vi "Resource Monitor.vi"() -> ()   [LabVIEW 2012]
doc: "Shows totals and availability for CPUs, hard drive, and memory resources."
uses:
  <vilib>/Utility/error.llb/DialogType.ctl
  <vilib>/nisyscfg/Close (Hardware).vi
  <vilib>/nisyscfg/Close (System).vi
  <resource>/objmgr/nisysapi.rc
  <vilib>/nisyscfg/nisyscfg.lvlib
panel:
  in  "Polling Interval":u32
  in  "User Name":string
  in  "Password":string
  in  "Target (localhost)":refnum<k21>="localhost"
  in  "stop":bool
  in  "System Properties":enum32{"CPU Usage", "Memory Usage"}(tab)
  out "CPU 0":u32[][](graph)
  out "CPU 2":u32[][](graph)
  out "CPU 3":u32[][](graph)
  out "CPU 1":u32[][](graph)
  out "CPU 4":u32[][](graph)
  out "CPU 5":u32[][](graph)
  out "CPU 6":u32[][](graph)
  out "CPU 7":u32[][](graph)
  out "Number of CPUs":i32
  out "Hard Drive Space Used (%)":dbl(slide) scale=0.0..100.0
  out "Memory":dbl[][](graph)
  out "Primary Hard Drive Available (MB)":dbl
  out "Total Physical Memory (MB)":u32
  out "Total Virtual Memory (MB)":u32
  out "Primary Hard Drive Capacity (MB)":u32
  # "Overview: Shows totals and availability for CPUs, hard drive, and memory resources. \nRequirements: NI System Configuration\nInstructions:\n1. Select your Target. Enter User Name and Password.\n2. Run the VI."
  # "Graphs will automatically populate with the number of cores detected on the computer. For systems with more then eight cores, only the first eight cores will be graphed in this example."
  # "NOTE: If values are 0, then the property is not supported by the specified Target."
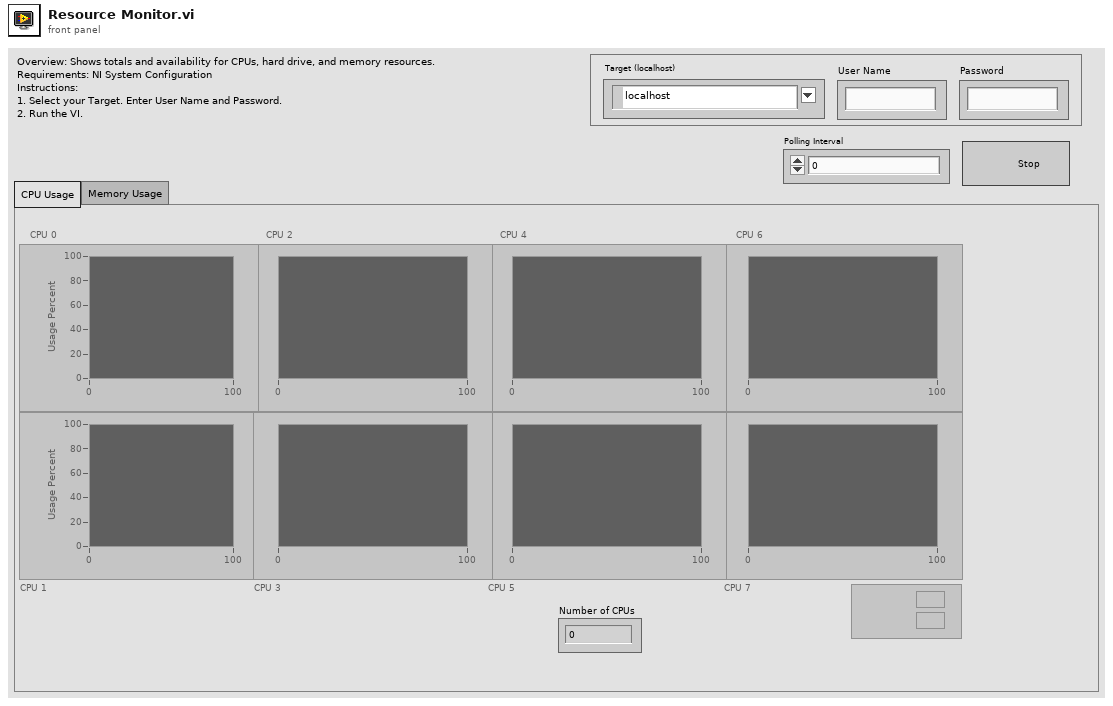
[diagram p1: front panel]
types:
  T1 = typedef "DialogType.ctl" = u16
  T2 = enum8{"Enabled", "Disabled", "Disabled and Grayed Out"}
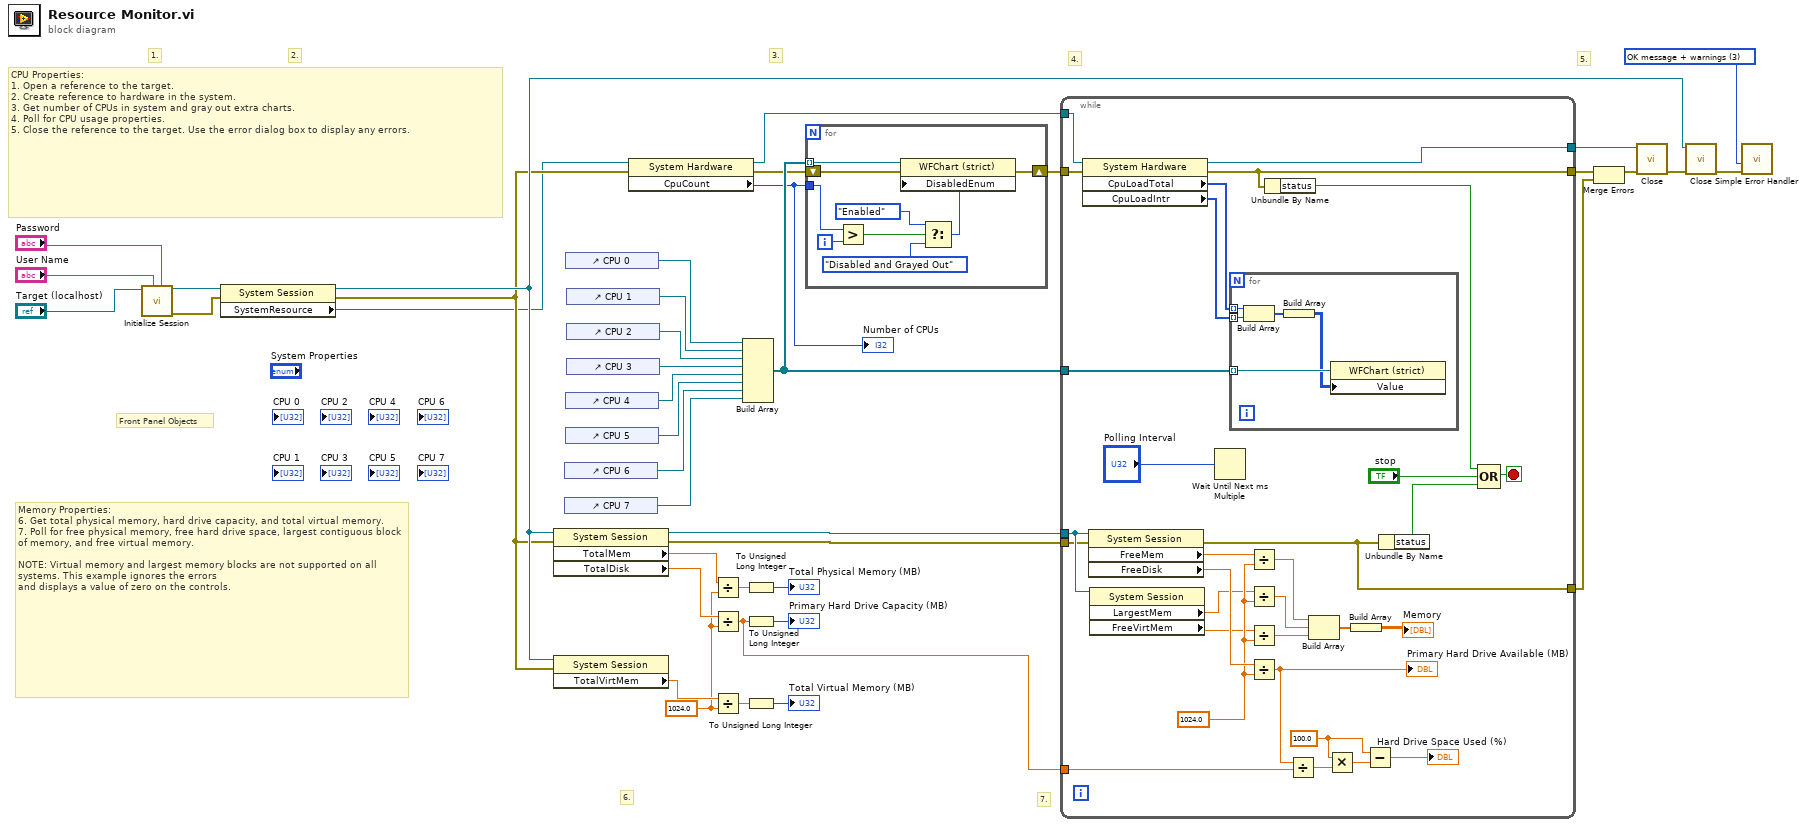
[diagram p0: block diagram]
diagram:
  w15 = T1 3 items=["no dialog", "OK message", "continue or stop message", "OK message + warnings", "continue/stop + warnings"] ("type of dialog (OK msg:1)")
  w23 = 1024.0
  # "2."
  # "Front Panel Objects"
  # "4."
  # "5."
  # "3."
  # "1."
  # "CPU Properties:\n1. Open a reference to the target.\n2. Create reference to hardware in the system.\n3. Get number of CPUs in system and gray out extra charts.\n4. Poll for CPU usage properties.\n5. Close the reference to the target. Use the error dialog box to display any errors."
  # "Memory Properties:\n6. Get total physical memory, hard drive capacity, and total virtual memory.\n7. Poll for free physical memory, free hard drive space, largest contiguous block of memory, and free virtual memory.\n\nNOTE: Virtual memory and largest memory blocks are not supported on all systems. This example ignores the errors\nand displays a value of zero on the controls."
  # "7."
  # "6."
  n1 = call <vilib>:"Initialize Session.vi"("Password"="Password", "User Name"="User Name", "Target (localhost)"="Target (localhost)") -> ("error out"=w8:errorcluster, "Session out"=w9:refnum<k21>)  [unwired: 7 in]
  n2 = property class="System Session"(reference=w9, error in=w8) -> (reference out=w7:refnum<k21>, error out=w6:errorcluster, "SystemResource"=w5:refnum<k20>)
  n3 = property class="System Session"(reference=w7, error in=w6) -> (reference out=w17:refnum<k21>, error out=w13:errorcluster, "TotalMem"=w26:dbl, "TotalDisk"=w25:dbl)
  n4 = property class="System Session"(reference=w7, error in=w6) -> ("TotalVirtMem"=w24:dbl)  [unwired: 2 out]
  n5 = control-ref of="CPU 6"() -> (w34:refnum<vi>)
  n6 = control-ref of="CPU 7"() -> (w27:refnum<vi>)
  n7 = control-ref of="CPU 0"() -> (w4:refnum<vi>)
  n8 = control-ref of="CPU 4"() -> (w36:refnum<vi>)
  n9 = control-ref of="CPU 5"() -> (w35:refnum<vi>)
  n10 = control-ref of="CPU 1"() -> (w39:refnum<vi>)
  n11 = control-ref of="CPU 2"() -> (w38:refnum<vi>)
  n12 = control-ref of="CPU 3"() -> (w37:refnum<vi>)
  n13 = property class="System Hardware"(reference=w5, error in=w6) -> (reference out=w40:refnum<k20>, error out=w32:errorcluster, "CpuCount"=w30:i32)
  "Number of CPUs" <- w30
  n14 = Divide(x=w26, y=w23) -> (x/y=w22:dbl)
  n15 = Divide(x=w25, y=w23) -> (x/y=w16:dbl)
  n16 = Divide(x=w24, y=w23) -> (x/y=w21:dbl)
  n17 = Build Array(w4, w39, w38, w37, w36, w35, w34, w27) -> (w33:refnum<vi>[])
  n18 = To Unsigned Long Integer(number=w22) -> (unsigned 32bit integer=→"Total Physical Memory (MB)":u32)
  n19 = To Unsigned Long Integer(number=w16) -> (unsigned 32bit integer=→"Primary Hard Drive Capacity (MB)":u32)
  n20 = To Unsigned Long Integer(number=w21) -> (unsigned 32bit integer=→"Total Virtual Memory (MB)":u32)
  n21 = for {
    tunnel: w33 -> [w49] mode=indexing
    shift-right: [w47] -> w31
    shift-left: w32 -> [w48]
    tunnel: w30 -> [w46]
    i -> [w45]
    n22 = Greater?(x=w46, y=w45) -> (0:w41:bool)
    n23 = Select(t=T2."Enabled" ("Disabled"), s=w41, f=T2."Disabled and Grayed Out" ("Disabled")) -> (s? t:f=w42:T2)
    n24 = property class="WFChart (strict)"(reference=w49, error in=w48, "DisabledEnum"=w42) -> (error out=w47:errorcluster)  [unwired: 1 out]
  }
  n25 = while {
    tunnel: [w80] -> w28
    tunnel: w40 -> [w79]
    tunnel: w31 -> [w78]
    tunnel: [w77] -> w12
    tunnel: w33 -> [w74]
    tunnel: w17 -> [w66]
    tunnel: w13 -> [w65]
    tunnel: [w61] -> w11
    tunnel: w16 -> [w57]
    stop <- w59 stop-if-true
    w52 = 100.0 ("y")
    w68 = 1024.0
    n26 = property class="System Hardware"(reference=w79, error in=w78) -> (reference out=w80:refnum<k20>, error out=w77:errorcluster, "CpuLoadTotal"=w75:u32[], "CpuLoadIntr"=w76:u32[])
    n27 = property class="System Session"(reference=w66, error in=w65) -> (error out=w61:errorcluster, "FreeMem"=w73:dbl, "FreeDisk"=w69:dbl)  [unwired: 1 out]
    n28 = property class="System Session"(reference=w66) -> ("LargestMem"=w55:dbl, "FreeVirtMem"=w56:dbl)  [unwired: 1 in, 2 out]
    n29 = Wait Until Next ms Multiple(millisecond multiple="Polling Interval") -> ()  [unwired: 1 out]
    n30 = for {
      tunnel: w76 -> [w84] mode=indexing
      tunnel: w75 -> [w85] mode=indexing
      tunnel: w74 -> [w82] mode=indexing
      n31 = Build Array(w85, w84) -> (w83:u32[])
      n32 = Build Array(w83) -> (w81:u32[][])
      n33 = property class="WFChart (strict)"(reference=w82, "Value"=w81) -> ()  [unwired: 1 in, 2 out]
    }
    n34 = Divide(x=w73, y=w68) -> (x/y=w71:dbl)
    n35 = Divide(x=w55, y=w68) -> (x/y=w70:dbl)
    n36 = Divide(x=w56, y=w68) -> (x/y=w67:dbl)
    n37 = Divide(x=w69, y=w68) -> (x/y=w58:dbl)
    "Primary Hard Drive Available (MB)" <- w58
    n38 = Unbundle By Name(w77) -> ("status"=w62:bool)
    n39 = Divide(x=w58, y=w57) -> (x/y=w51:dbl)
    n40 = Build Array(w71, w70, w67) -> (w72:dbl[])
    n41 = Multiply(x=w52, y=w51) -> (x*y=w54:dbl)
    n42 = Build Array(w72) -> (→"Memory":dbl[][])
    n43 = Subtract(x=w52, y=w54) -> (x-y=→"Hard Drive Space Used (%)":dbl)
    n44 = Unbundle By Name(w61) -> ("status"=w63:bool)
    n45 = Compound Arithmetic op=OR(w62, "stop", w63) -> (w59:bool)
  }
  n46 = Merge Errors(w12, w11) -> (w10:errorcluster)
  n47 = call-poly <vilib>:"Close.vi"("error in (no error)"=w10, "Resource in"=w28) -> ("error out"=w29:errorcluster)  [unwired: 9 in]
  n48 = call-poly <vilib>:"Close.vi"("error in (no error)"=w29, "Session in"=w7) -> ("error out"=w14:errorcluster)  [unwired: 9 in]
  n49 = call <vilib>:"Simple Error Handler.vi"("type of dialog (OK msg:1)"=w15, "error in (no error)"=w14) -> ()  [unwired: 3 in, 5 out]
